vi "sv_Peak View Harmonics (1 Ch).vi"(7 "harmonic units":T7(ring), 8 "error in (no error)":errorcluster, 9 "spectrum info":T1={"channel name"="", "description"="", "x-axis units"=0, "spectral info"={"spectrum type"=enum."Power [Magnitude^2]", "linear/dB"=enum."linear", "window"=0, "window size"=0, "FFT size"=0}, "engineering units"=0, "custom label"="", "dB reference [EU]"=0.0, "peak units"=enum."rms", "weighting filter"=0, "spectral density?"=FALSE, "unit label"="", "spectrum skewed?"=FALSE, "complimentary spectrum units"=enum."none"} {"x-axis units" items=["Time (s)"=0, "Frequency-CB (Hz)"=1, "Frequency-CPB (Hz)"=1248, "Frequency-Arbitrary (Hz)"=2357, "Quefrency (s)"=2, "Revolutions (rev)"=3, "Order"=4, "Speed (RPM)"=11, "Speed (rad/s)"=21, "Index"=65535]; "weighting filter" items=["Linear", "A-weighting", "B-weighting", "C-weighting", "ITU-R 468-4", "Dolby", "CCITT", "C-message", "Wb", "Wc", "Wd", "We", "Wf", "Wh", "Wj", "Wk", "Wm", "AES17 20 kHz lowpass", "AES17 40 kHz lowpass", "AES17 20 kHz highpass", "AES17 40 kHz highpass"]; "dB reference [EU]" format="%.2f"; "engineering units" items=["custom..."=0, "V"=1, "A"=21, "C"=30, "pC"=31, "s"=32, "-"=29, "Pa"=2, "N"=20, "g"=3, "m/s^2"=4, "m/s"=5, "m"=6, "mm/s"=12, "mm"=13, "micron/s"=14, "micron"=15, "in/s^2"=7, "in/s"=8, "in"=9, "mil/s"=10, "mil"=11, "rad/s^2"=16, "rad/s"=17, "rad"=18, "deg/s^2"=26, "deg/s"=27, "deg"=28, "RPM"=22, "cycle/s^2"=23, "Hz"=24, "cycle"=25, "strain"=19]; "spectral info"."window" items=["None "=0, "Hanning"=1, "Hamming"=2, "Blackman-Harris"=3, "Exact Blackman"=4, "Blackman"=5, "Flat Top"=6, "4 Term B-Harris "=7, "7 Term B-Harris"=8, "Low Sidelobe"=9, "Force - Exponential"=10, "Gaussian"=62]}, 10 "fundamental amplitude [EU pk]":dbl format="%.2f", 11 "harmonic amplitude [EU pk]":dbl format="%.2f") -> (0 "error out":errorcluster, 3 "converted harmonic amplitude":dbl=nan format="%.2f", 5 "unit label":string)   [LabVIEW 2017, in "SoundVib_Distortion.lvlib"]
uses:
  <vilib>/addons/Sound and Vibration/svt_Distortion/SoundVib_Distortion.lvlib
  <vilib>/addons/_NISVFA/_Shared subVIs/Controls/svc_Spectrum Info.ctl
  <vilib>/addons/_NISVFA/_Shared subVIs/Controls/svc_X-Axis Units.ctl
  <vilib>/addons/_NISVFA/_Shared subVIs/Controls/svc_Spectrum Type.ctl
  <vilib>/addons/_NISVFA/_Shared subVIs/Controls/svc_Engineering Units Text Ring.ctl
  <vilib>/addons/_NISVFA/_Shared subVIs/Controls/svc_Weighting Filter Text Ring.ctl
  <vilib>/addons/_NISVFA/_Shared subVIs/Controls/svc_Complimentary Spectrum Units.ctl
  <vilib>/addons/_NISVFA/_Shared subVIs/Common/svc_Get Weighting Enum and Labels.vi
  <vilib>/addons/_NISVFA/_Shared subVIs/Common/svc_Unit Label Lexical Class.vi
  <vilib>/addons/_NISVFA/_Shared subVIs/Common/svc_Engineering Units to Unit Label.vi
  <vilib>/addons/_NISVFA/_Shared subVIs/Common/svc_Format Value (DBL).vi
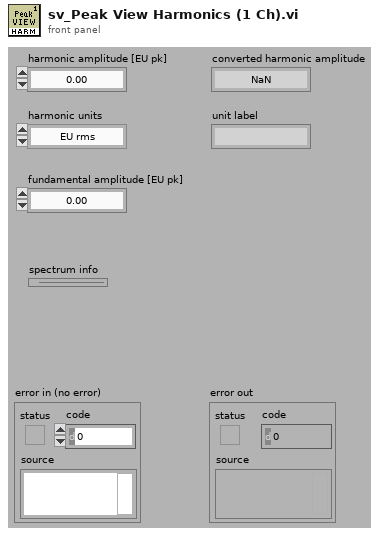
[diagram p1: front panel]
types:
  T1 = typedef "svc_Spectrum Info.ctl" = cluster{"channel name":string, "description":string, "x-axis units":T2, "spectral info":cluster{"spectrum type":T3, "linear/dB":enum16{"linear", "dB"}, "window":u16, "window size":i32, "FFT size":i32}, "engineering units":T4, "custom label":string, "dB reference [EU]":dbl, "peak units":enum16{"rms", "peak", "peak-peak"}, "weighting filter":T5, "spectral density?":bool, "unit label":string, "spectrum skewed?":bool, "complimentary spectrum units":T6}
  T2 = typedef "svc_X-Axis Units.ctl" = u16
  T3 = typedef "svc_Spectrum Type.ctl" = enum16{"FFT Spectrum [complex]", "Amplitude [Magnitude]", "Power [Magnitude^2]", "Cross Spectrum [complex]", "Frequency Response [Complex]"}
  T4 = typedef "svc_Engineering Units Text Ring.ctl" = u16
  T5 = typedef "svc_Weighting Filter Text Ring.ctl" = u16
  T6 = typedef "svc_Complimentary Spectrum Units.ctl" = enum16{"none", "radians", "degrees", "cycles", "imaginary"}
  T7 = enum16{"EU rms", "EU peak", "EU peak-peak", "dB ref fund"}
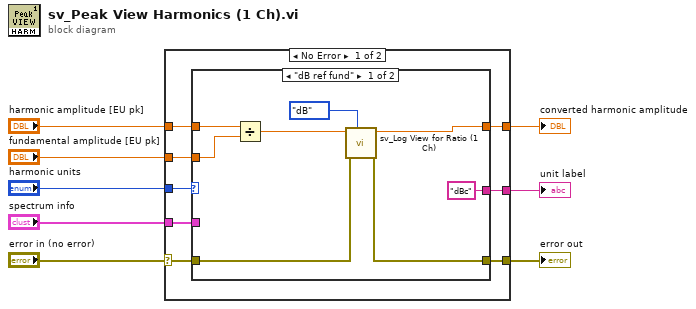
[diagram p0: block diagram]
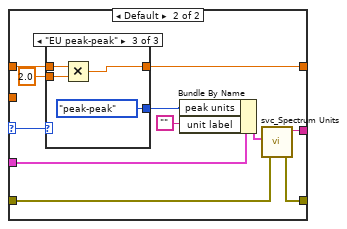
[diagram p2: hidden frame]
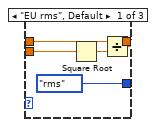
[diagram p3: hidden frame]
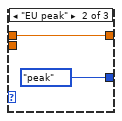
[diagram p4: hidden frame]
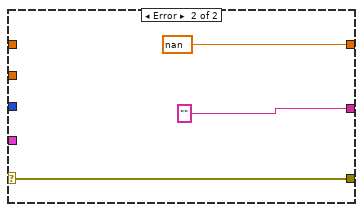
[diagram p5: hidden frame]
diagram:
  n1 = case shown="No Error" "error in (no error)" {
    selector: "error in (no error)" -> [w12 w47]
    tunnel: [w13 ""] -> w8
    tunnel: [w16 nan ("peak amplitude [EU pk]")] -> w7
    tunnel: "harmonic amplitude [EU pk]" -> [w15 _]
    tunnel: "harmonic units" -> [w10 _]
    tunnel: [w11 w47] -> w3
    tunnel: "spectrum info" -> [w14 _]
    tunnel: "fundamental amplitude [EU pk]" -> [w9 _]
    frame No Error {
      n2 = case shown="\"dB ref fund\"" w10 {
        selector: w10 -> [_ w29]
        tunnel: [w18 w34] -> w16
        tunnel: w15 -> [w23 w33]
        tunnel: w14 -> [_ w28]
        tunnel: ["dBc" ("unit label") w32] -> w13
        tunnel: w12 -> [w21 w31]
        tunnel: [w20 w30] -> w11
        tunnel: w9 -> [w24 _]
        frame "dB ref fund" {
          n3 = Divide(x=w23, y=w24) -> (x/y=w22:dbl)
          n4 = call <vilib>:"sv_Log View for Ratio (1 Ch).vi"("ratio units"=enum16{"dB", "linear ratio", "%"}."dB", "error in (no error)"=w21, "linear ratio"=w22) -> ("error out"=w20:errorcluster, "converted ratio"=w18:dbl)  [unwired: 6 in, 1 out]
        }
        frame Default {
          n5 = case shown="\"EU peak-peak\"" w29 {
            tunnel: w33 -> [w40 w42 w45]
            tunnel: [w37 w42 w44] -> w34
            tunnel: 2.0 ("y") -> [w38 _ w46]
            tunnel: [enum16{"rms", "peak", "peak-peak"}."rms" ("peak units") enum16{"rms", "peak", "peak-peak"}."peak" ("peak units") enum16{"rms", "peak", "peak-peak"}."peak-peak" ("peak units")] -> w26
            frame "EU rms", Default {
              n6 = Square Root(x=w38) -> (sqrt(x)=w39:dbl)
              n7 = Divide(x=w40, y=w39) -> (x/y=w37:dbl)
            }
            frame "EU peak" {
            }
            frame "EU peak-peak" {
              n8 = Multiply(x=w45, y=w46) -> (x*y=w44:dbl)
            }
          }
          n9 = Bundle By Name(cluster=w28, "peak units"=w26, "unit label"="") -> (w27:T1)
          n10 = call <vilib>:"svc_Spectrum Units.vi"("error in (no error)"=w31, "spectrum info in"=w27) -> ("error out"=w30:errorcluster, "unit label"=w32:string)  [unwired: 2 in, 2 out]
        }
      }
    }
    frame Error {
    }
  }
  "unit label" <- w8
  "converted harmonic amplitude" <- w7
  "error out" <- w3
